vi "loadControlsFromTarget.vi"(8 "error in (no error)":errorcluster, 9 "ConnectionData":T1, 10 "ControlsToLoad":refnum<vi>[](array[refnum]), 11 "ConfigXMLControls":T2) -> (0 "error out":errorcluster)   [LabVIEW 2016]
uses:
  ConfigXMLControl.ctl
  General/CorePluginInfo.ctl
  General/RemoteFiles/connectionData.ctl
panel:
  # "Fetches the current file from the target, saves it to ${CONFIG_HOME}\\targetDownloads\\<date>\\ConfigOnTarget_<time>.xml"
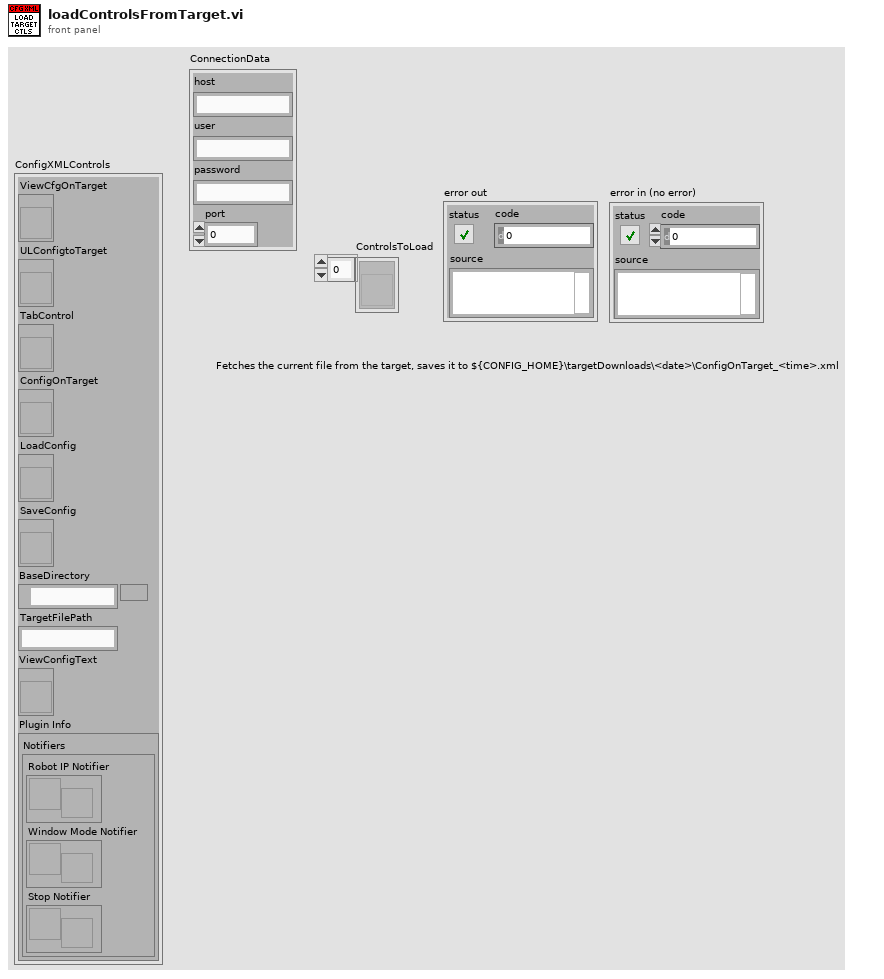
[diagram p1: front panel]
types:
  T1 = typedef "connectionData.ctl" = cluster{"host":string, "user":string, "password":string, "port":u16}
  T2 = typedef "ConfigXMLControl.ctl" = cluster{"ViewCfgOnTarget":refnum<vi>, "ULConfigtoTarget":refnum<vi>, "TabControl":refnum<vi>, "ConfigOnTarget":refnum<vi>, "LoadConfig":refnum<vi>, "SaveConfig":refnum<vi>, "BaseDirectory":path, "TargetFilePath":string, "ViewConfigText":refnum<vi>, "Plugin Info":T3}
  T3 = typedef "CorePluginInfo.ctl" = cluster{"Notifiers":cluster{"Robot IP Notifier":refnum<notifier>, "Window Mode Notifier":refnum<notifier>, "Stop Notifier":refnum<notifier>}}
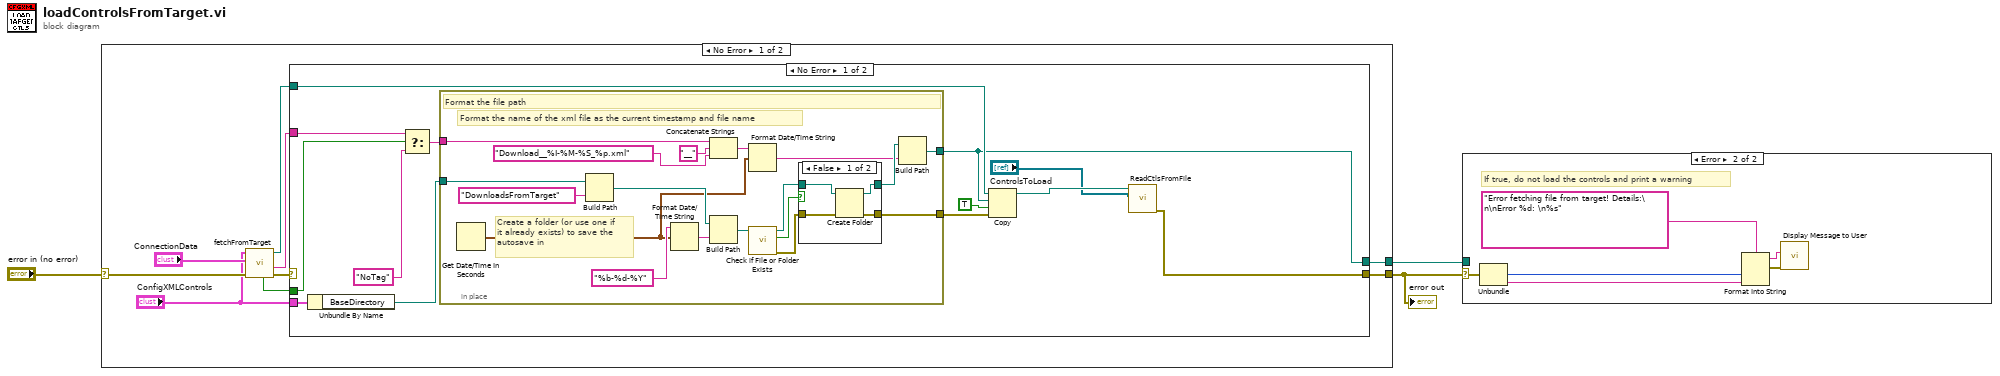
[diagram p0: block diagram]
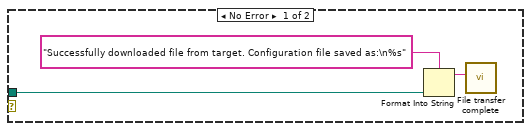
[diagram p2: hidden frame]
diagram:
  n1 = case shown="No Error" "error in (no error)" {
    selector: "error in (no error)" -> [w8 w50]
    tunnel: [w12 w50] -> w2
    tunnel: [w4 _] -> w1
    frame No Error {
      n2 = call "fetchFromTarget.vi"("error in (no error)"=w8, "ConnectionData"="ConnectionData", "ConfigXMLControls"="ConfigXMLControls") -> ("error out"=w10:errorcluster, "nameMessageOut"=w6:string, "path out"=w9:path, "NameTagFound"=w5:bool)  [unwired: 4 in, 1 out]
      n3 = case shown="No Error" w10 {
        selector: w10 -> [_ w49]
        tunnel: [w13 w49] -> w12
        tunnel: w9 -> [w22 _]
        tunnel: "ConfigXMLControls" -> [w25 _]
        tunnel: w6 -> [w19 _]
        tunnel: w5 -> [w20 _]
        tunnel: [w16 _] -> w4
        frame No Error {
          n4 = Unbundle By Name(w25) -> ("BaseDirectory"=w23:path)
          n5 = Select(t=w19, s=w20, f="NoTag") -> (s? t:f=w18:string)
          n6 = in-place {
            in-place-border: [w34] -> w16
            in-place-border: w23 -> [w33]
            in-place-border: [w32] -> w21
            in-place-border: w18 -> [w26]
            # "Format the name of the xml file as the current timestamp and file name"
            # "Create a folder (or use one if\nit already exists) to save the\nautosave in"
            # "Format the file path"
            n7 = Get Date/Time In Seconds() -> (seconds since 1Jan1904=w28:timestamp)
            n8 = Build Path(base path=w33, name or relative path="DownloadsFromTarget") -> (appended path=w41:path)
            n9 = Format Date/Time String(time format string (%c)="%b-%d-%Y", seconds (now)=w28) -> (date/time string=w40:string)  [unwired: 1 in]
            n10 = Concatenate Strings(w26, "__" ("string"), "Download__%I-%M-%S_%p.xml" ("time format string (%c)")) -> (w29:string)
            n11 = Build Path(base path=w41, name or relative path=w40) -> (appended path=w39:path)
            n12 = Format Date/Time String(time format string (%c)=w29, seconds (now)=w28) -> (date/time string=w27:string)  [unwired: 1 in]
            n13 = call <vilib>:"Check if File or Folder Exists.vi"("path"=w39) -> ("error out"=w35:errorcluster, "file or folder exists?"=w38:bool, "dup path"=w37:path)  [unwired: 8 in]
            n14 = case shown="False" w38 {
              tunnel: w37 -> [w47 w48]
              tunnel: [w46 w48] -> w36
              tunnel: [w45 _] -> w32
              tunnel: w35 -> [w44 _]
              frame False {
                n15 = Create Folder(path (use dialog)=w47, error in=w44) -> (created path=w46:path, error out=w45:errorcluster)  [unwired: 1 in, 1 out]
              }
              frame True {
              }
            }
            n16 = Build Path(base path=w36, name or relative path=w27) -> (appended path=w34:path)
          }
          n17 = Copy(8:w21, 9:TRUE ("overwrite (F)"), 10:w16, 11:w22) -> (3:w15:path)  [unwired: 1 in, 2 out]
          n18 = call "ReadCtlsFromFile.vi"("ControlsToLoad"="ControlsToLoad", "selected path"=w15) -> ("error out"=w13:errorcluster)  [unwired: 9 in]
        }
        frame Error {
        }
      }
    }
    frame Error {
    }
  }
  "error out" <- w2
  n19 = case shown="Error" w2 {
    selector: w2 -> [_ w54]
    tunnel: w1 -> [w51 _]
    frame No Error {
      n20 = Format Into String(format string="Successfully downloaded file from target. Configuration file saved as:\n%s", w51) -> (resulting string=w52:string)  [unwired: 2 in, 1 out]
      n21 = call "File transfer complete"("Message"=w52) -> ()  [unwired: 9 in, 2 out]
    }
    frame Error {
      # "If true, do not load the controls and print a warning"
      n22 = Unbundle(w54) -> ("code"=w55:i32, "source"=w56:string)  [unwired: 1 out]
      n23 = Format Into String(format string="Error fetching file from target! Details:\n\nError %d: \n%s" ("Message"), w55, w56) -> (resulting string=w58:string, error out=w59:errorcluster)  [unwired: 2 in]
      n24 = call "Display Message to User"("error in (no error)"=w59, "Message"=w58) -> ()  [unwired: 8 in, 2 out]
    }
  }
